vi "decimal_to_digits_arr.vi"() -> ()   [LabVIEW 2019]
panel:
  out "Array":dbl[](array[numeric])
  in  "Numeric":dbl
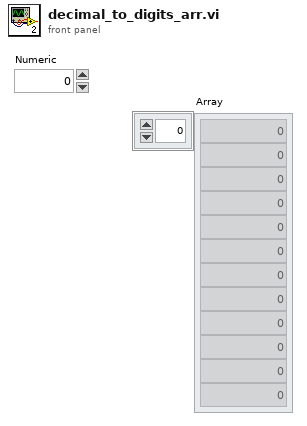
[diagram p1: front panel]
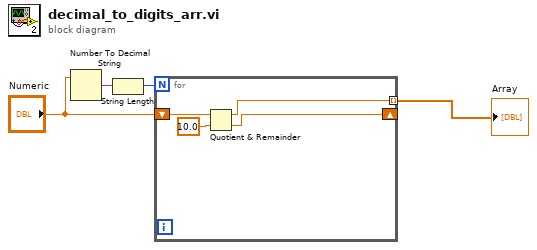
[diagram p0: block diagram]
diagram:
  n1 = Number To Decimal String(number="Numeric") -> (decimal integer string=w4:string)  [unwired: 1 in]
  n2 = String Length(string=w4) -> (length=w3:i32)
  n3 = for {
    N: w3 -> [_]
    shift-right: [w6] -> _
    shift-left: "Numeric" -> [w8]
    tunnel: [w5] -> w1 mode=indexing
    n4 = Quotient & Remainder(x=w8, y=10.0) -> (x-y*floor(x/y)=w5:dbl, floor(x/y)=w6:dbl)
  }
  "Array" <- w1
